vi "MS SQL_InRFID_STN60.vi"(5 "OP30_VERIFY_STN":T1, 6 "RFID":string, 8 "error in (no error)":errorcluster, 11 "Ref in":T2={"MS SQL Connection"=refnum, "UDL File"=path "", "Time"="", "DCODE"="", "WIP+1"=0, "MC No?"=0, "POKAYOKE?"=FALSE, "Expected Result"="", "Result [Status]"="", "Clock"=0.0, "RFID"="", "WIP Queue"=refnum, "TS Parameter"={"ProfitCenterCode"="", "LineCode"="", "WorkOrderNumber"="", "Model"="", "Model_with_Prefix"="", "VendorCode"="", "SetParameterDateCode"="", "PokaYoke"=0, "Target"=1, "Live_DateCode"="", "CustomerPartNumber"="", "Hand"="", "sBarcode"=FALSE, "FCA"=0, "Ent_Stamp"=timestamp(0 s since 1904-01-01), "STS_CD"=0.0}, "Data_Queue"=[], "RFID Serial No."=""} {"TS Parameter"."FCA" format="%01d"; "TS Parameter"."Target" min=1 max=100000; "TS Parameter"."PokaYoke" min=0 max=1}) -> (0 "error out":errorcluster, 1 "Message":picture, 3 "Ref Out":T2={"MS SQL Connection"=refnum, "UDL File"=path "", "Time"="", "DCODE"="", "WIP+1"=0, "MC No?"=0, "POKAYOKE?"=FALSE, "Expected Result"="", "Result [Status]"="", "Clock"=0.0, "RFID"="", "WIP Queue"=refnum, "TS Parameter"={"ProfitCenterCode"="", "LineCode"="", "WorkOrderNumber"="", "Model"="", "Model_with_Prefix"="", "VendorCode"="", "SetParameterDateCode"="", "PokaYoke"=0, "Target"=1, "Live_DateCode"="", "CustomerPartNumber"="", "Hand"="", "sBarcode"=FALSE, "FCA"=0, "Ent_Stamp"=timestamp(0 s since 1904-01-01), "STS_CD"=0.0}, "Data_Queue"=[], "RFID Serial No."=""} {"TS Parameter"."FCA" format="%01d"; "TS Parameter"."Target" min=1 max=100000; "TS Parameter"."PokaYoke" min=0 max=1})   [LabVIEW 2020]
uses:
  Controls/TD SQL.ctl
  <vilib>/addons/database/Connection.llb/Conn ObjectReference.ctl
  Controls/WIP_State.ctl
  Controls/TS_Parameter.ctl
  <vilib>/addons/database/NI_Database_API.lvlib
panel:
  out "resulting string":string
  # "OP80"
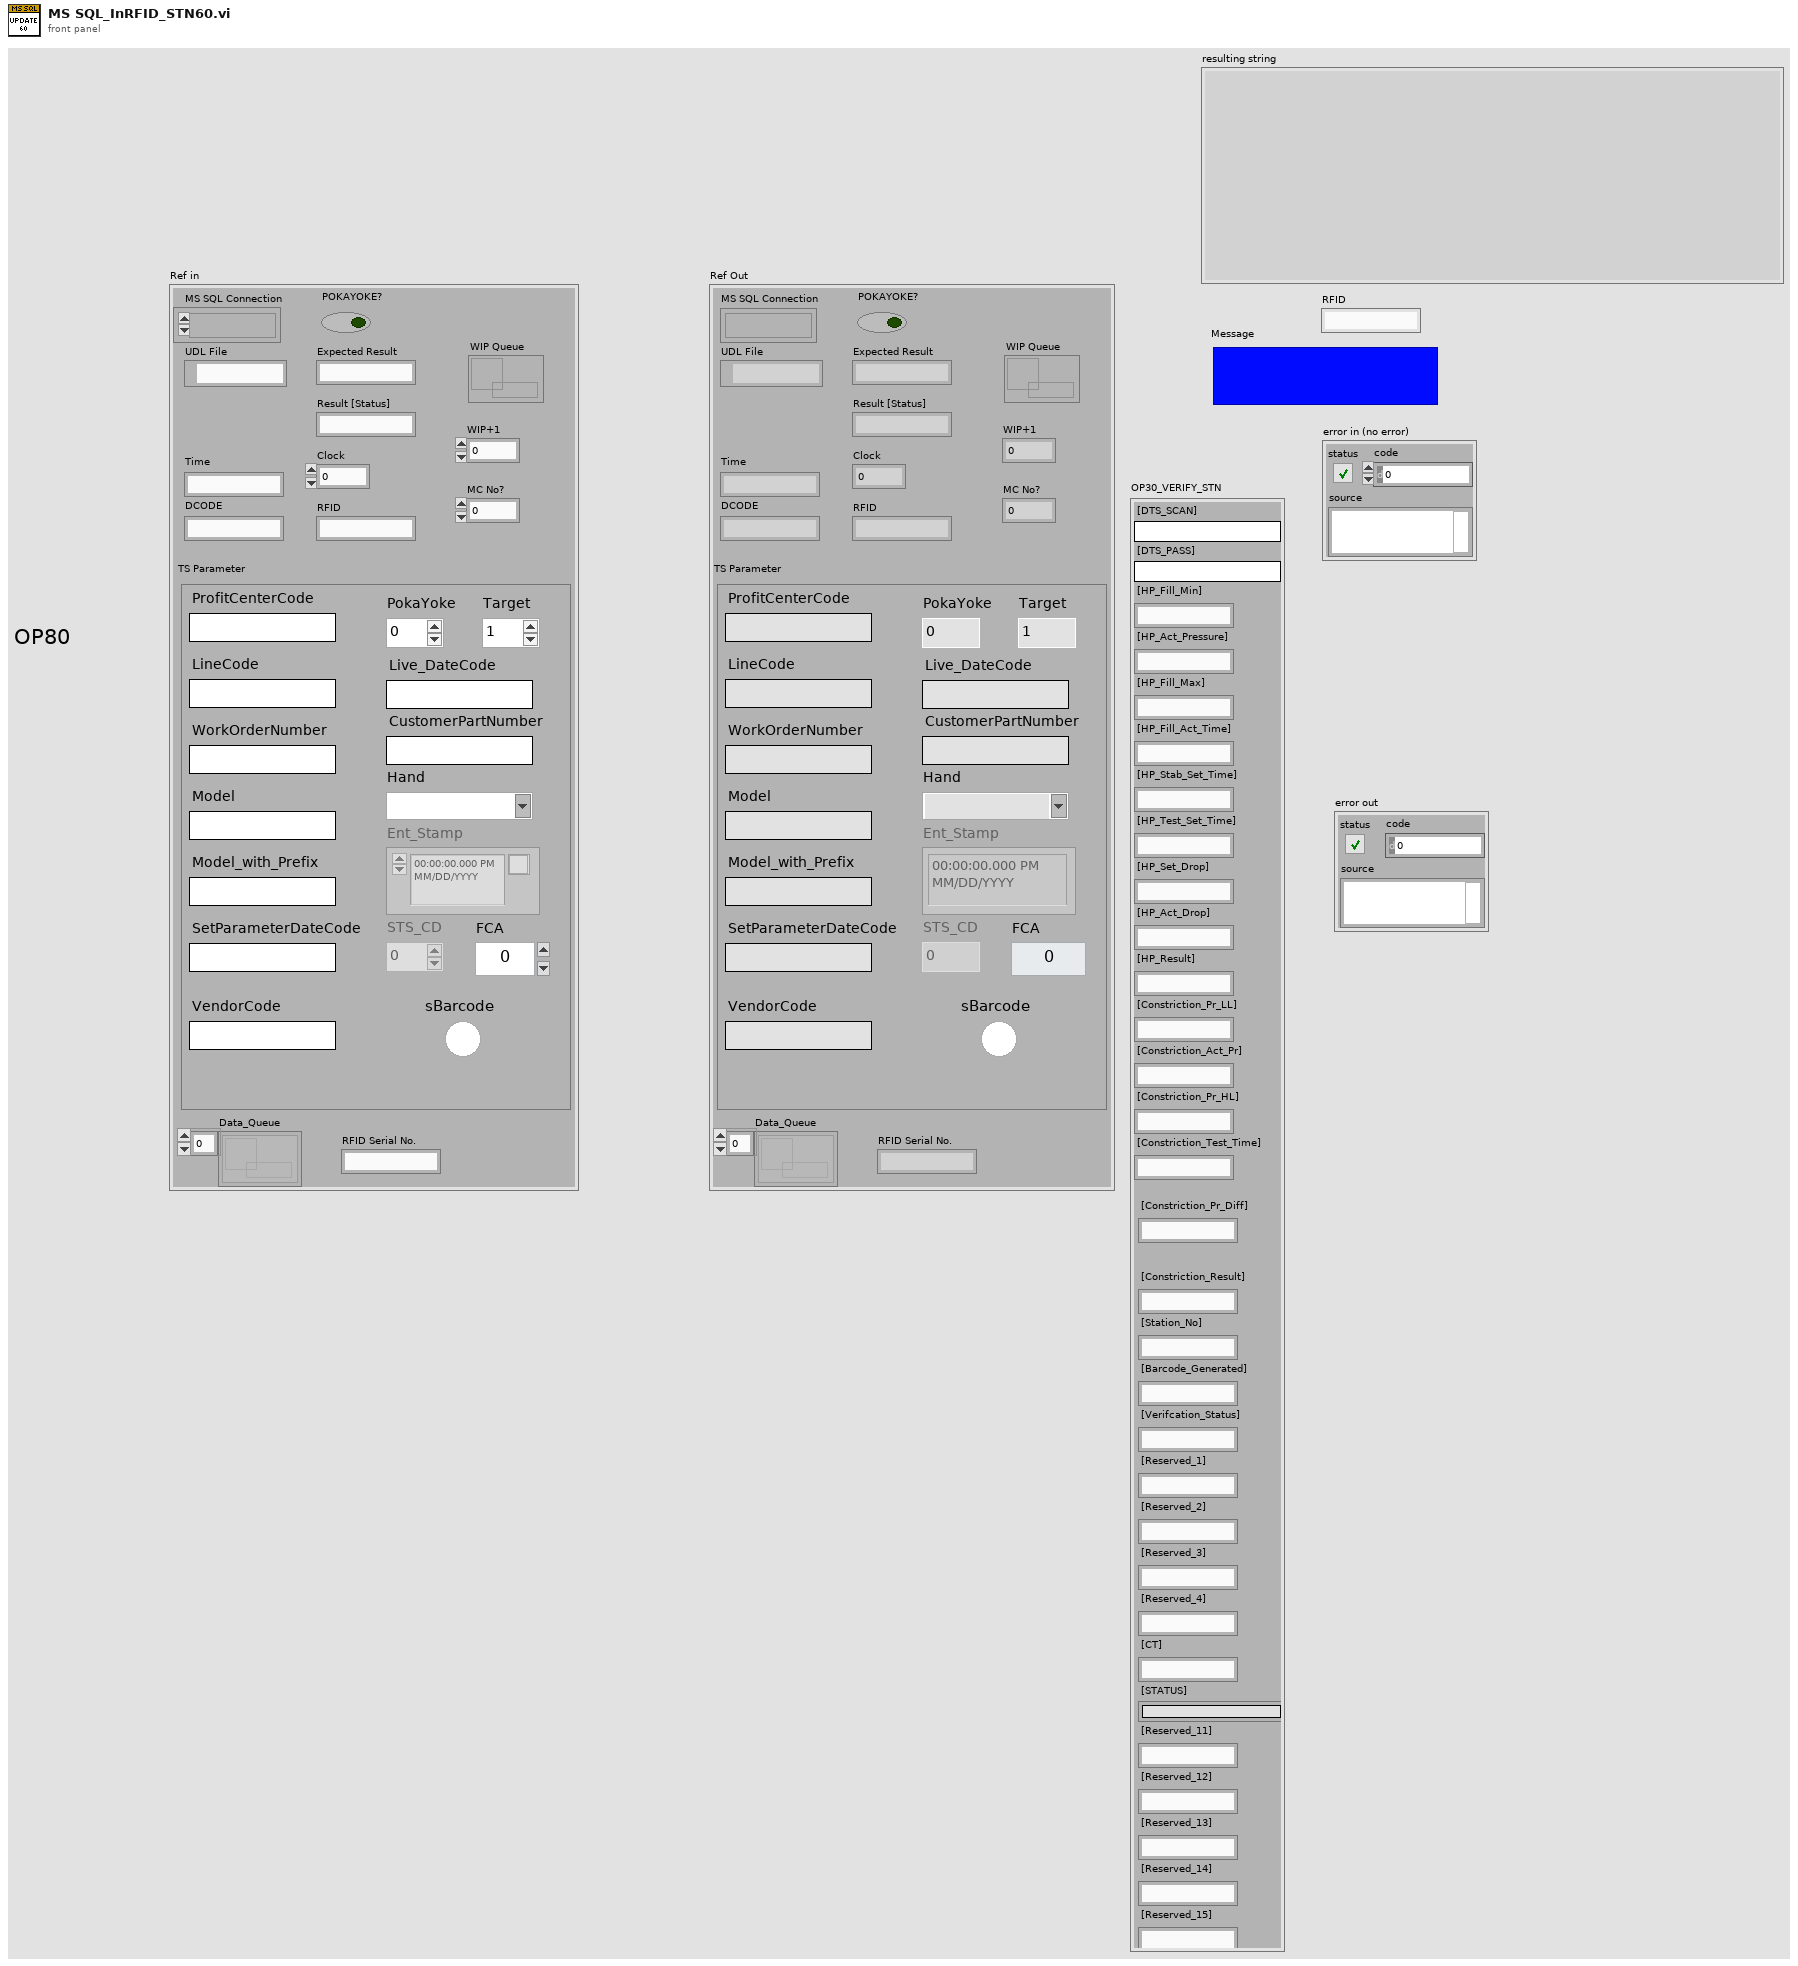
[diagram p1: front panel]
types:
  T1 = cluster{"[DTS_SCAN]":string, "[DTS_PASS]":string, "[HP_Fill_Min]":string, "[HP_Act_Pressure]":string, "[HP_Fill_Max]":string, "[HP_Fill_Act_Time]":string, "[HP_Stab_Set_Time]":string, "[HP_Test_Set_Time]":string, "[HP_Set_Drop]":string, "[HP_Act_Drop]":string, "[HP_Result]":string, "[Constriction_Pr_LL]":string, "[Constriction_Act_Pr]":string, "[Constriction_Pr_HL]":string, "[Constriction_Test_Time]":string, "[Constriction_Pr_Diff]":string, "[Constriction_Result]":string, "[Station_No]":string, "[Barcode_Generated]":string, "[Verifcation_Status]":string, "[Reserved_1]":string, "[Reserved_2]":string, "[Reserved_3]":string, "[Reserved_4]":string, "[CT]":string, "[STATUS]":string, "[Reserved_11]":string, "[Reserved_12]":string, "[Reserved_13]":string, "[Reserved_14]":string, "[Reserved_15]":string}
  T2 = typedef "TD SQL.ctl" = cluster{"MS SQL Connection":T3, "UDL File":path, "Time":string, "DCODE":string, "WIP+1":i64, "MC No?":i32, "POKAYOKE?":bool, "Expected Result":string, "Result [Status]":string, "Clock":dbl, "RFID":string, "WIP Queue":refnum<queue>, "TS Parameter":T4, "Data_Queue":refnum<queue>[], "RFID Serial No.":string}
  T3 = typedef "NI_Database_API.lvlib/Conn ObjectReference.ctl" = refnum<k1>
  T4 = typedef "TS_Parameter.ctl" = cluster{"ProfitCenterCode":string, "LineCode":string, "WorkOrderNumber":string, "Model":string, "Model_with_Prefix":string, "VendorCode":string, "SetParameterDateCode":string, "PokaYoke":i32, "Target":i32, "Live_DateCode":string, "CustomerPartNumber":string, "Hand":string, "sBarcode":bool, "FCA":i32, "Ent_Stamp":timestamp, "STS_CD":dbl}
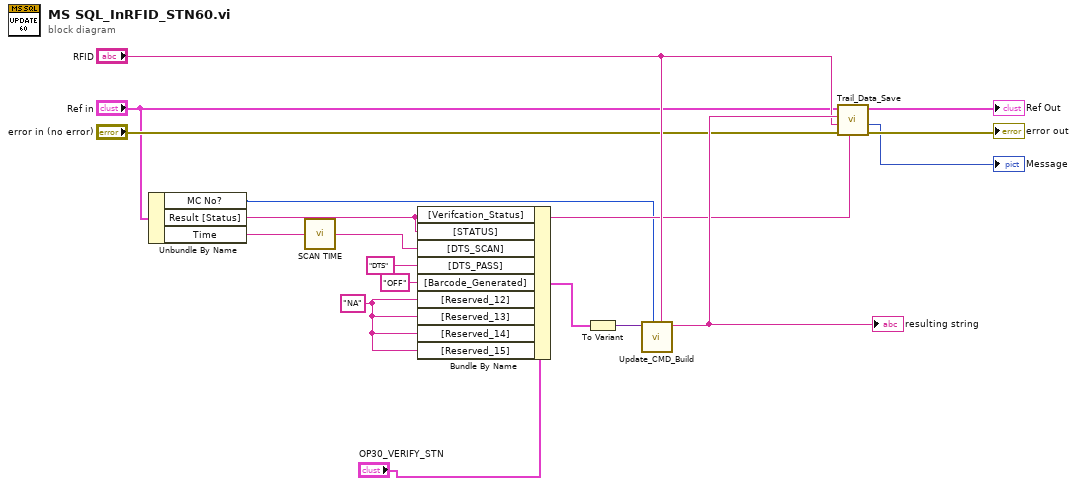
[diagram p0: block diagram]
diagram:
  w2 = "NA" ("[Reserved_1]")
  n1 = Unbundle By Name("Ref in") -> ("MC No?"=w4:i32, "Result [Status]"=w5:string, "Time"=w9:string)
  n2 = call "SCAN TIME.vi"("Time in"=w9) -> ("Time out"=w16:string)
  n3 = Bundle By Name(cluster="OP30_VERIFY_STN", "[Verifcation_Status]"=w5, "[STATUS]"=w5, "[DTS_SCAN]"=w16, "[DTS_PASS]"="DTS", "[Barcode_Generated]"="OFF", "[Reserved_12]"=w2, "[Reserved_13]"=w2, "[Reserved_14]"=w2, "[Reserved_15]"=w2) -> (w7:T1)
  n4 = To Variant(anything=w7) -> (Variant=w17:variant)
  n5 = call "Update_CMD_Build.vi"("RFID"="RFID", "Machine No"=w4, "Variant"=w17) -> ("Update Query"=w14:string)  [unwired: 5 in, 1 out]
  "resulting string" <- w14
  n6 = call "Trail_Data_Save.vi"("Status"=w5, "error in (no error)"="error in (no error)", "RFID"="RFID", "Query"=w14, "Ref in"="Ref in") -> ("error out"=→"error out":errorcluster, "Message"=→"Message":picture, "Ref Out"=→"Ref Out":T2)  [unwired: 1 in, 1 out]
